vi "Dequeue Frame.vi"(8 "error in":errorcluster) -> (0 "error out":errorcluster, 3 "Data":string[][](array[string]))   [LabVIEW 2025, in "CAN-LIN Raw Bus Capture.lvclass"]
uses:
  CAN-LIN Raw Bus Capture.lvclass
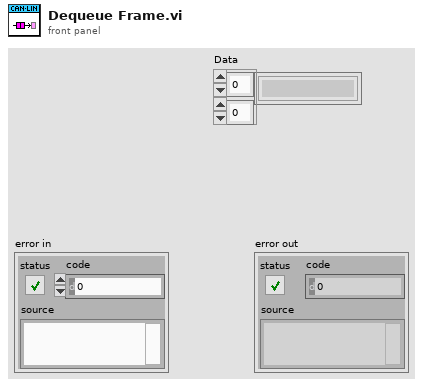
[diagram p1: front panel]
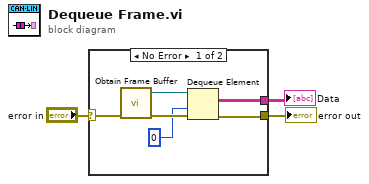
[diagram p0: block diagram]
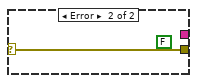
[diagram p2: hidden frame]
diagram:
  n1 = case shown="No Error" "error in" {
    selector: "error in" -> [w9 w10]
    tunnel: [w5 w10] -> w2
    tunnel: [w4 _] -> w1
    frame No Error {
      n2 = call "Obtain Frame Buffer.vi"("error in"=w9) -> ("error out"=w8:errorcluster, "queue out"=w7:refnum<queue>)  [unwired: 9 in]
      n3 = Dequeue Element(queue=w7, timeout in ms (-1)=0, error in (no error)=w8) -> (element=w4:string[][], error out=w5:errorcluster)  [unwired: 2 out]
    }
    frame Error {
      (unwired) FALSE ("overflow?")
    }
  }
  "error out" <- w2
  "Data" <- w1
